vi "Stop Core.vi"(10 "final error code":i32, 11 "Vision in":refnum<class "Vision.lvclass">) -> (3 "Vision out":refnum<class "Vision.lvclass">)   [LabVIEW 2019, in "Vision.lvlib" / "Vision.lvclass"]
doc: "(<B>Filename</B>: Actor Framework.lvlib:Actor.lvclass:Stop Core.vi)\n\nDefines what the actor does before it stops. Use the <B>final error code</B> input to determine whether the actor shut down in response to an error.\n\nBy default, this method passes the Stop message along to all auto-stop nested actors. A descendant class may override this method to define additional behavior, such as shutting down any processes the actor initiated in its override of the Actor Core method."
uses:
  Vision.lvclass
  Vision.lvclass/Vision.ctl
  <vilib>/ActorFramework/Actor/Actor.lvclass
  <vilib>/vision/driver/NI_Vision_Acquisition_Software.lvlib
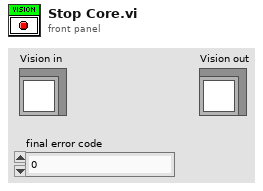
[diagram p1: front panel]
types:
  T1 = typedef "IMAQdx.ctl" = refnum<k21>
  T2 = typedef "IMAQ Image.ctl" = refnum<image>
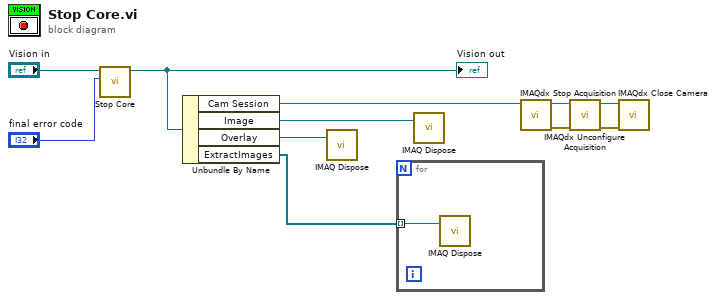
[diagram p0: block diagram]
diagram:
  n1 = call-parent "Stop Core.vi"("final error code"="final error code", "Actor in"="Vision in") -> ("Actor out"=w9:refnum<class "Vision.lvclass">)  [unwired: 9 in]
  "Vision out" <- w9
  n2 = Unbundle By Name(w9) -> ("Cam Session"=w2:T1, "Image"=w8:T2, "Overlay"=w1:T2, "ExtractImages"=w7:T2[])
  n3 = call "IMAQ Dispose"("Image"=w1) -> ()  [unwired: 5 in, 1 out]
  n4 = for {
    tunnel: w7 -> [w12] mode=indexing
    n5 = call "IMAQ Dispose"("Image"=w12) -> ()  [unwired: 5 in, 1 out]
  }
  n6 = call "IMAQ Dispose"("Image"=w8) -> ()  [unwired: 5 in, 1 out]
  n7 = call <vilib>:"IMAQdx Stop Acquisition.vi"("Session In"=w2) -> ("error out"=w3:errorcluster, "Session Out"=w4:T1)  [unwired: 1 in, 8 out]
  n8 = call <vilib>:"IMAQdx Unconfigure Acquisition.vi"("error in"=w3, "Session In"=w4) -> ("error out"=w6:errorcluster, "Session Out"=w5:T1)  [unwired: 8 out]
  n9 = call <vilib>:"IMAQdx Close Camera.vi"("error in"=w6, "Session In"=w5) -> ()  [unwired: 10 out]
